vi "0816039.vi"() -> ()   [LabVIEW 2021]
uses:
  <vilib>/Utility/miscctls.llb/LVDateTimeRec.ctl
  <vilib>/Analysis/NI_AALBase.lvlib
panel:
  in  "stop":bool
  out "date time rec":T1
  out "XY Graph":cluster{dbl[], dbl[]}[](graph)
  in  "phase(degrees)":dbl format="%0.2f"
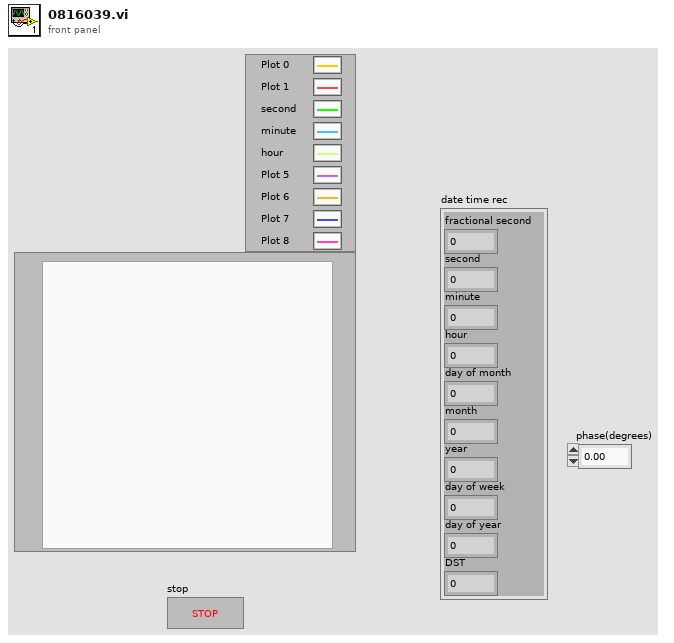
[diagram p1: front panel]
types:
  T1 = typedef "LVDateTimeRec.ctl" = cluster{"fractional second":dbl, "second":i32, "minute":i32, "hour":i32, "day of month":i32, "month":i32, "year":i32, "day of week":i32, "day of year":i32, "DST":i32}
  T2 = cluster{"Sinusoidal Pattern":dbl[], "Sinusoidal Pattern":dbl[]}
  T3 = cluster{"Sinusoidal Pattern":dbl[], "Sinusoidal Pattern":dbl[]}[]
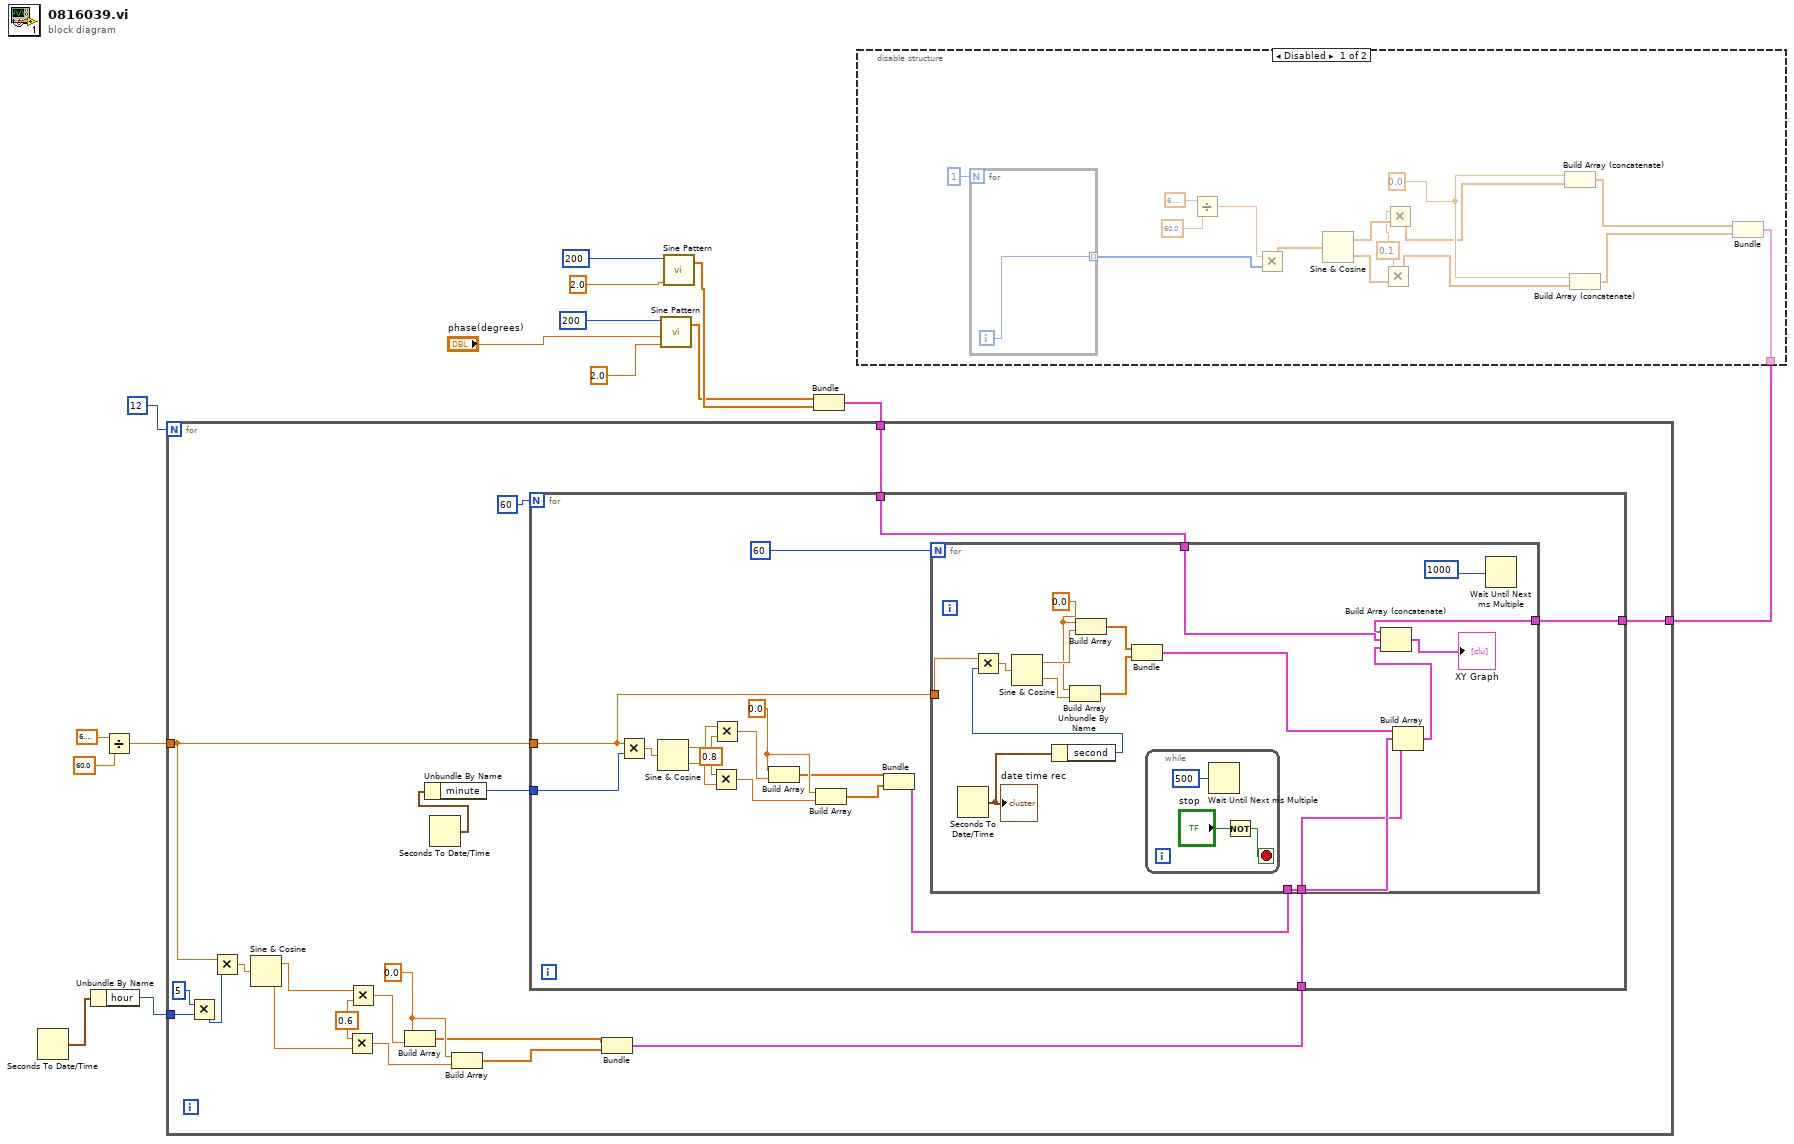
[diagram p0: block diagram]
diagram:
  n1 = Seconds To Date/Time() -> (date time rec=w4:T1)  [unwired: 2 in]
  n2 = Unbundle By Name(w4) -> ("hour"=w3:i32)
  n3 = Divide(x=6.283185307179586, y=60.0) -> (x/y=w5:dbl)
  n4 = call <vilib>:"Sine Pattern.vi"("cycles"=2.0, "phase(degrees)"="phase(degrees)", "samples"=200) -> ("Sinusoidal Pattern"=w9:dbl[])  [unwired: 1 in, 1 out]
  n5 = call <vilib>:"Sine Pattern.vi"("cycles"=2.0, "samples"=200) -> ("Sinusoidal Pattern"=w10:dbl[])  [unwired: 2 in, 1 out]
  n6 = Bundle("Sinusoidal Pattern"=w9, "Sinusoidal Pattern"=w10) -> (w8:T2)  [unwired: 1 in]
  n7 = disable-structure shown="Disabled" {
    disable-tunnel: [w19 _] -> w1
    frame Disabled {
      w16 = 0.1
      w28 = 0.0 ("element")
      n8 = for {
        N: 1 -> [_]
        tunnel: [w31] -> w21 mode=indexing
        i -> [w31]
      }
      n9 = Divide(x=6.283185307179586, y=60.0) -> (x/y=w20:dbl)
      n10 = Multiply(x=w20, y=w21) -> (x*y=w22:dbl[])
      n11 = Sine & Cosine(0:w22) -> (1:w30:dbl[], 2:w29:dbl[])
      n12 = Multiply(x=w16, y=w29) -> (x*y=w17:dbl[])
      n13 = Multiply(x=w16, y=w30) -> (x*y=w18:dbl[])
      n14 = Build Array (concatenate)(w28, w18) -> (w27:dbl[])
      n15 = Build Array (concatenate)(w28, w17) -> (w26:dbl[])
      n16 = Bundle(w27, w26) -> (w19:cluster{dbl[], dbl[]})  [unwired: 1 in]
    }
    frame Enabled {
    }
  }
  n17 = for {
    N: 12 -> [_]
    tunnel: w8 -> [w50]
    tunnel: w5 -> [w47]
    tunnel: w3 -> [w36]
    tunnel: w1 -> [w32]
    w41 = 0.0 ("element")
    w46 = 0.6 ("y")
    n18 = Multiply(x=5, y=w36) -> (x*y=w34:i32)
    n19 = Multiply(x=w47, y=w34) -> (x*y=w48:dbl)
    n20 = Sine & Cosine(0:w48) -> (1:w43:dbl, 2:w42:dbl)
    n21 = Multiply(x=w46, y=w42) -> (x*y=w44:dbl)
    n22 = Multiply(x=w43, y=w46) -> (x*y=w45:dbl)
    n23 = Build Array(w41, w45) -> (w40:dbl[])
    n24 = Seconds To Date/Time() -> (date time rec=w37:T1)  [unwired: 2 in]
    n25 = Unbundle By Name(w37) -> ("minute"=w35:i32)
    n26 = Build Array(w41, w44) -> (w39:dbl[])
    n27 = Bundle(w40, w39) -> (w38:cluster{dbl[], dbl[]})  [unwired: 1 in]
    n28 = for {
      N: 60 -> [_]
      tunnel: w50 -> [w55]
      tunnel: w47 -> [w54]
      tunnel: w38 -> [w53]
      tunnel: w35 -> [w52]
      tunnel: w32 -> [w51]
      w60 = 0.0 ("element")
      w62 = 0.8 ("y")
      n29 = Multiply(x=w54, y=w52) -> (x*y=w65:dbl)
      n30 = Sine & Cosine(0:w65) -> (1:w64:dbl, 2:w63:dbl)
      n31 = Multiply(x=w62, y=w63) -> (x*y=w59:dbl)
      n32 = Multiply(x=w64, y=w62) -> (x*y=w61:dbl)
      n33 = Build Array(w60, w61) -> (w58:dbl[])
      n34 = Build Array(w60, w59) -> (w57:dbl[])
      n35 = Bundle(w58, w57) -> (w56:cluster{dbl[], dbl[]})  [unwired: 1 in]
      n36 = for {
        N: 60 -> [_]
        tunnel: w54 -> [w82]
        tunnel: w56 -> [w75]
        tunnel: w55 -> [w72]
        tunnel: w53 -> [w70]
        tunnel: w51 -> [w67]
        w79 = 0.0 ("element")
        n37 = Seconds To Date/Time() -> (date time rec=w69:T1)  [unwired: 2 in]
        "date time rec" <- w69
        n38 = Unbundle By Name(w69) -> ("second"=w68:i32)
        n39 = Multiply(x=w82, y=w68) -> (x*y=w83:dbl)
        n40 = Sine & Cosine(0:w83) -> (1:w81:dbl, 2:w80:dbl)
        n41 = Build Array(w79, w80) -> (w77:dbl[])
        n42 = Build Array(w79, w81) -> (w78:dbl[])
        n43 = Bundle(w78, w77) -> (w76:cluster{dbl[], dbl[]})  [unwired: 1 in]
        n44 = while {
          stop <- w84 stop-if-true
          n45 = Wait Until Next ms Multiple(millisecond multiple=u32 500) -> ()  [unwired: 1 out]
          n46 = Not(x="stop") -> (.not. x?=w84:bool)
        }
        n47 = Build Array(w76, w75, w70) -> (w73:cluster{dbl[], dbl[]}[])
        n48 = Build Array (concatenate)(w67, w72, w73) -> (→"XY Graph":T3)
        n49 = Wait Until Next ms Multiple(millisecond multiple=u32 1000) -> ()  [unwired: 1 out]
      }
    }
  }
